vi "FileDialog.vi"(8 "Error In":errorcluster, 11 "File Path Control In":path) -> (0 "Error Out":errorcluster, 2 "Valid File Path":bool, 3 "File Path Control Out":path)   [LabVIEW 2018]
doc: "This VI sets the optional strings in the rings based on what is available in the configuration INI files."
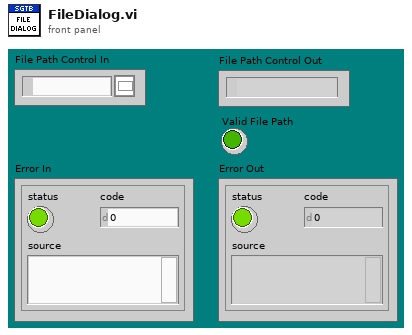
[diagram p1: front panel]
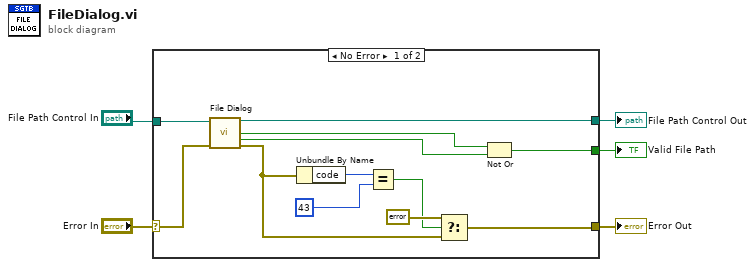
[diagram p0: block diagram]
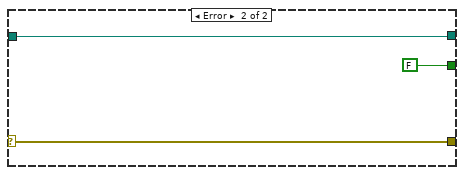
[diagram p2: hidden frame]
diagram:
  n1 = case shown="No Error" "Error In" {
    selector: "Error In" -> [w9 w20]
    tunnel: "File Path Control In" -> [w10 w19]
    tunnel: [w8 w20] -> w4
    tunnel: [w7 w19] -> w2
    tunnel: [w6 FALSE] -> w1
    frame No Error {
      n2 = call "File Dialog"("start path"=w10, "error in"=w9) -> ("selected path"=w7:path, "exists"=w12:bool, "cancelled"=w11:bool, "error out"=w16:errorcluster)  [unwired: 10 in]
      n3 = Unbundle By Name(w16) -> ("code"=w14:i32)
      n4 = Equal?(x=w14, y=43 ("code")) -> (x = y?=w13:bool)
      n5 = Select(t=errorcluster {"status"=FALSE, "code"=0, "source"=""} ("error out"), s=w13, f=w16) -> (s? t:f=w8:errorcluster)
      n6 = Not Or(1:w11, 2:w12) -> (0:w6:bool)
    }
    frame Error {
    }
  }
  "Error Out" <- w4
  "File Path Control Out" <- w2
  "Valid File Path" <- w1
